vi "Test ID Generated for Data without ID.vi"(8 "error in (no error)":errorcluster, 11 "Test Case In":refnum<class "Debug Log Test.lvclass">) -> (0 "error out":errorcluster, 3 "Test Case Out":refnum<class "Debug Log Test.lvclass">)   [LabVIEW 2020, in "Debug Log Test.lvclass"]
uses:
  Debug Log Test.lvclass
  C:/Program Files (x86)/National Instruments/LabVIEW 2020/vi.lib/Astemes/LUnit/Test Case.lvclass
  source/Debug Log/Debug Log.lvclass
  source/Debug Data/Raw Debug Data.ctl
  source/Debug Log/Debug Log.lvclass/Debug Log.ctl
  source/Debug Data/Debug Data.lvclass/Debug Data.ctl
  <vilib>/Astemes/LUnit/Test Case.lvclass/Test Case.ctl
  <vilib>/Astemes/LUnit/LUnit Assertion Result.lvclass/LUnit Assertion Result.ctl
  <vilib>/Astemes/LUnit/LUnit Test Case Result.lvclass/LUnit Test Case Result.ctl
  <vilib>/Astemes/LUnit/LUnit Method Result.lvclass/LUnit Method Result.ctl
  e110ba72-c4f9-4de7-bf05-3ebd5ee4e4e5.vi
  source/Debug Log/Read Unfiltered Log Content.vi
  <vilib>/Astemes/LUnit/Palette/Pass.vi
  <vilib>/Astemes/LUnit/Palette/Fail.vi
  <vilib>/Astemes/LUnit/Compare Variants.vi
  <vilib>/Astemes/LUnit/Describe Comparison.vi
  <vilib>/Astemes/LUnit/Set Assertion Type.vi
  <vilib>/Astemes/LUnit/Add test result.vi
  <vilib>/Astemes/LUnit/LUnit Write Passed.vi
  <vilib>/Astemes/LUnit/LUnit Write Message.vi
  <vilib>/Astemes/LUnit/LUnit Write Description.vi
  <vilib>/Astemes/LUnit/Variant to string.vi
  <vilib>/Astemes/LUnit/LUnit Write Assertion Type.vi
  <vilib>/Astemes/LUnit/LUnit Record Assertion Result.vi
  <vilib>/Astemes/LUnit/LUnit Aggregate Assertion Results.vi
  <vilib>/Astemes/LUnit/Assertion Result/LUnit Read Status.vi
  <vilib>/Astemes/LUnit/LUnit Read Message.vi
  <vilib>/Astemes/LUnit/LUnit Read Description.vi
  <vilib>/Astemes/LUnit/Method Result/LUnit Merge Status.vi
  <vilib>/Astemes/LUnit/LUnit Concatenate result strings.vi
  <vilib>/Utility/Data Type/Get Type Information.vi
  <vilib>/Utility/LVClass/Get LV Class Name.vi
  <vilib>/Astemes/LUnit/LUnit Assertion Result.lvclass
  source/Filter/Filter.lvclass
  Debug Log Test.lvclass/Debug Log Test.ctl
  source/Debug Data/Debug Data.lvclass
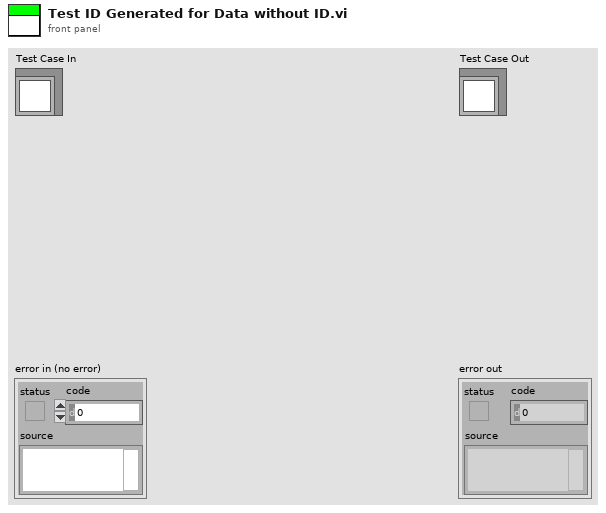
[diagram p1: front panel]
types:
  T1 = typedef "Debug Data.lvclass/Raw Debug Data.ctl" = cluster{"Action":string, "Call Chain":string, "Process":string, "Message":string, "Message Data":variant, "Time":dbl}
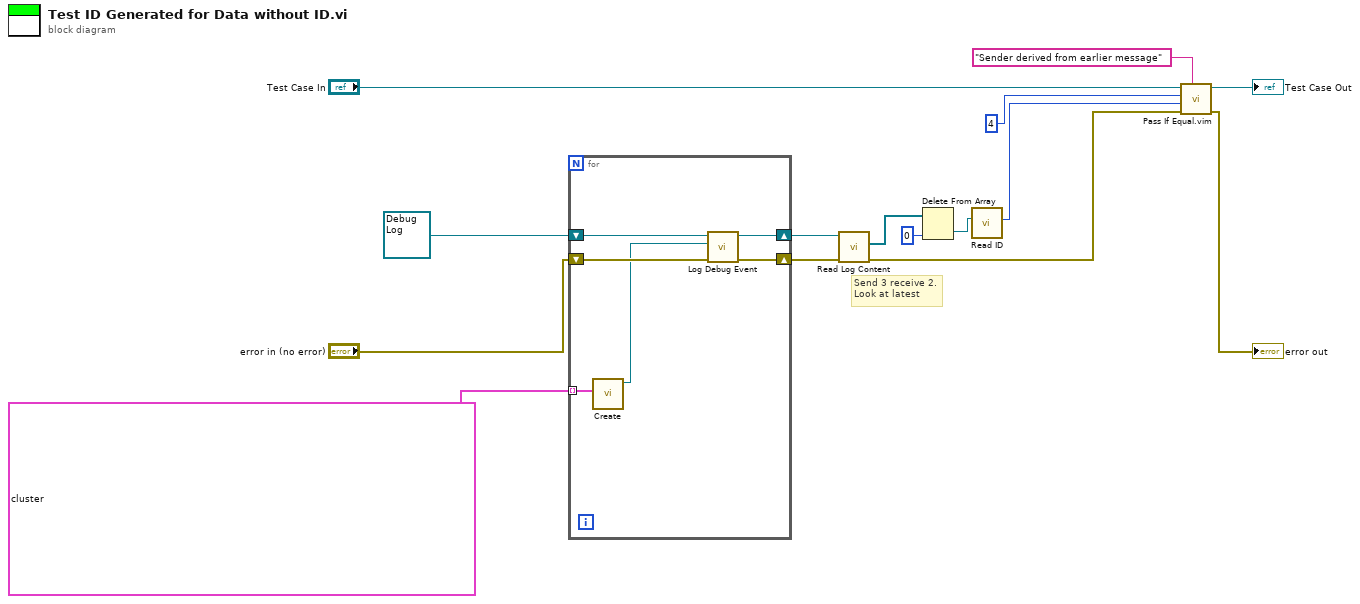
[diagram p0: block diagram]
diagram:
  # "Send 3 receive 2.\nLook at latest"
  n1 = for {
    tunnel: T1[] [{"Action"="Send", "Call Chain"="Test.vi", "Process"="", "Message"="asd", "Message Data"=variant, "Time"=0.0}, {"Action"="Send", "Call Chain"="Test.vi", "Process"="Process 1", "Message"="asd", "Message Data"=variant, "Time"=0.0}, {"Action"="Send", "Call Chain"="Test.vi", "Process"="Process 1", "Message"="asd", "Message Data"=variant, "Time"=0.0}, {"Action"="Receive", "Call Chain"="TF.lvlib:Process.lvclass:Handle Messages.vi:1960001", "Process"="Process 1", "Message"="asd", "Message Data"=variant, "Time"=0.0}, {"Action"="Receive", "Call Chain"="TF.lvlib:Process.lvclass:Handle Messages.vi:1960001", "Process"="Process 1", "Message"="asd", "Message Data"=variant, "Time"=0.0}] ("Debug Data Cluster") -> [w17] mode=indexing
    shift-right: [w20] -> w11
    shift-left: refnum<class "Debug Log.lvclass"> refnum ("Debug Log.lvclass") -> [w21]
    shift-right: [w18] -> w10
    shift-left: "error in (no error)" -> [w19]
    n2 = call "Create.vi"("Debug Data Cluster"=w17) -> ("Debug Data out"=w16:refnum<class "Debug Data.lvclass">)  [unwired: 9 in, 1 out]
    n3 = call "Log Debug Event.vi"("error in (no error)"=w19, "Debug Data.lvclass"=w16, "Debugger in"=w21) -> ("error out"=w18:errorcluster, "Debugger out"=w20:refnum<class "Debug Log.lvclass">)  [unwired: 7 in]
  }
  n4 = call "Read Log Content.vi"("error in (no error)"=w10, "Debug Log In"=w11) -> ("error out"=w13:errorcluster, "Data Log"=w4:refnum<class "Debug Data.lvclass">[])  [unwired: 7 in, 1 out]
  n5 = Delete From Array(array=w4, index=0) -> (deleted portion=w3:refnum<class "Debug Data.lvclass">)  [unwired: 1 in, 1 out]
  n6 = call "Read ID.vi"("Debug Data in"=w3) -> ("ID"=w2:u32)  [unwired: 9 in, 1 out]
  n7 = call "Pass If Equal.vim"("Description"="Sender derived from earlier message", "error in (no error)"=w13, "Actual"=w2, "Expected"=u32 4 ("size(s)"), "LUnit Test Case In"="Test Case In") -> ("error out"=→"error out":errorcluster, "LUnit Test Case Out"=→"Test Case Out":refnum<class "Debug Log Test.lvclass">)  [unwired: 5 in]
